vi "_importProcessBar.vi"(1 "Target IP":string="10.144.7.147", 3 "ProfileSrcPath":string[](array[string]), 5 "user name":string="admin", 7 "password":string="nigel", 11 "error in (no error)":errorcluster, 12 "importTarget?":bool=TRUE, 14 "importHost?":bool) -> (4 "hostResult":i32[](array[numeric]), 6 "targetResult":i32[](array[numeric]), 15 "error out":errorcluster)   [LabVIEW 2019, in "SEECD System Explorer.lvlib"]
uses:
  SEECD System Explorer.lvlib
panel:
  out "Transferring....":u8(slide) caption="Importing the profiles to the host computer" scale=0.0..57.0 scale format="%.6f"
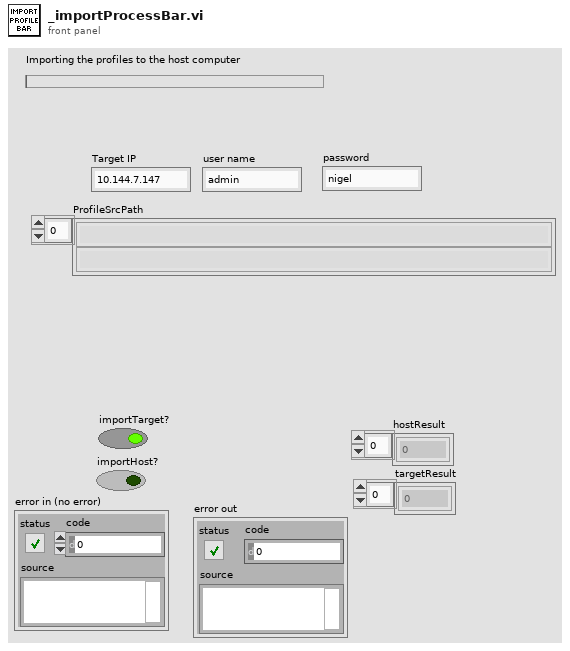
[diagram p1: front panel]
types:
  T1 = typedef "_profileImport.ctl" = cluster{"ddSrcPath":string, "ddDestPath":string, "result":i32, "isNIDDProfile":bool}
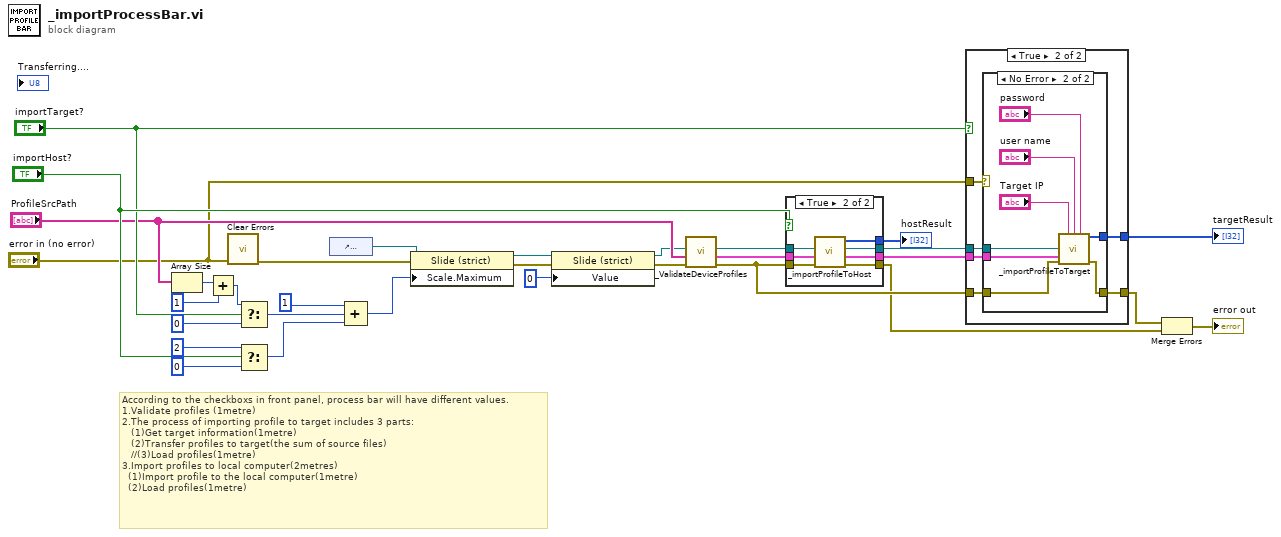
[diagram p0: block diagram]
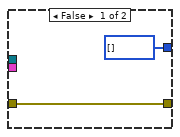
[diagram p2: hidden frame]
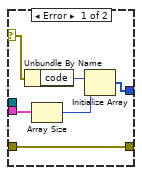
[diagram p3: hidden frame]
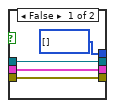
[diagram p4: hidden frame]
diagram:
  # "According to the checkboxs in front panel, process bar will have different values.\n1.Validate profiles (1metre)\n2.The process of importing profile to target includes 3 parts:\n   (1)Get target information(1metre)\n   (2)Transfer profiles to target(the sum of source files)\n   //(3)Load profiles(1metre)\n3.Import profiles to local computer(2metres)\n  (1)Import profile to the local computer(1metre)\n  (2)Load profiles(1metre)"
  n1 = Array Size(array="ProfileSrcPath") -> (size(s)=w29:i32)
  n2 = Add(x=w29, y=1) -> (x+y=w27:i32)
  n3 = call <vilib>:"Clear Errors.vi"("error in (no error)"="error in (no error)") -> ("error out"=w3:errorcluster)  [unwired: 5 in, 1 out]
  n4 = Select(t=w27, s="importTarget?", f=0) -> (s? t:f=w25:i32)
  n5 = Select(t=2, s="importHost?", f=0) -> (s? t:f=w24:i32)
  n6 = control-ref of="Transferring...."() -> (w19:refnum<vi>)
  n7 = Compound Arithmetic op=ADD(1 ("value"), w25, w24) -> (w22:i32)
  n8 = property on="Property Node" class="Slide (strict)"(reference=w19, error in=w3, "Scale.Maximum"=w22) -> (reference out=w20:refnum<vi>, error out=w13:errorcluster)
  n9 = property on="Property Node" class="Slide (strict)"(reference=w20, error in=w13, "Value"=u8 0 ("Transferring....")) -> (reference out=w7:refnum<vi>, error out=w8:errorcluster)
  n10 = call "_ValidateDeviceProfiles.vi"("error in (no error)"=w8, "ddSrcPath"="ProfileSrcPath", "reference in"=w7) -> ("error out"=w15:errorcluster, "profileImport"=w18:T1[], "reference out"=w17:refnum<vi>)  [unwired: 6 in]
  n11 = case shown="True" "importHost?" {
    tunnel: [i32[] [] ("result out") w42] -> w1
    tunnel: w18 -> [w33 w41]
    tunnel: w17 -> [w34 w36]
    tunnel: [w34 w40] -> w16
    tunnel: w15 -> [w32 w39]
    tunnel: [w33 w38] -> w14
    tunnel: [w32 w37] -> w10
    frame False {
    }
    frame True {
      n12 = call <resource>:"_importProfileToHost.vi"("error in"=w39, "profileImport"=w41, "reference in"=w36) -> ("error out"=w37:errorcluster, "profileImport out"=w38:T1[], "reference out"=w40:refnum<vi>, "result out"=w42:i32[])  [unwired: 4 in]
    }
  }
  "hostResult" <- w1
  n13 = case shown="True" "importTarget?" {
    tunnel: [i32[] [] ("result out") w50] -> w31
    tunnel: w16 -> [_ w49]
    tunnel: w15 -> [w43 w48]
    tunnel: w14 -> [_ w47]
    tunnel: "error in (no error)" -> [_ w46]
    tunnel: [w43 w45] -> w9
    frame False {
    }
    frame True {
      n14 = case shown="No Error" w46 {
        selector: w46 -> [w51 _]
        tunnel: [w55 w64] -> w50
        tunnel: w49 -> [_ w57]
        tunnel: w48 -> [w53 w63]
        tunnel: w47 -> [w56 w59]
        tunnel: [w53 w58] -> w45
        frame Error {
          n15 = Unbundle By Name(w51) -> ("code"=w52:i32)
          n16 = Array Size(array=w56) -> (size(s)=w54:i32)
          n17 = Initialize Array(w52, w54) -> (w55:i32[])
        }
        frame No Error {
          n18 = call <resource>:"_importProfileToTarget.vi"("Target IP"="Target IP", "user name"="user name", "password"="password", "reference in"=w57, "profileImport"=w59, "error in"=w63) -> ("result out"=w64:i32[], "error out"=w58:errorcluster)  [unwired: 6 in, 2 out]
        }
      }
    }
  }
  "targetResult" <- w31
  n19 = Merge Errors(w9, w10) -> (→"error out":errorcluster)
